vi "Write.vi"(5 "TDMS Channel in":refnum<class "Channel.lvclass">, 8 "error in (no error)":errorcluster, 9 "Channel Properties":refnum<class "Variant.lvclass">, 10 "Array Data":refnum<class "Generic Array Data.lvclass">, 11 "Channel Name":string) -> (0 "error out":errorcluster, 3 "TDMS Channel out":refnum<class "Channel.lvclass">)   [LabVIEW 2020, in "TDMS.lvlib" / "Channel.lvclass"]
doc: "Write Channel Name, Data and Properties."
uses:
  Channel.lvclass
  PPL/HDH.Data.Generic.lvlibp/Generic Data/Generic Array Data/Generic Array Data.lvclass
  PPL/HDH.Data.Generic.lvlibp/Generic Data/Variant/Variant.lvclass
  Channel.lvclass/Channel.ctl
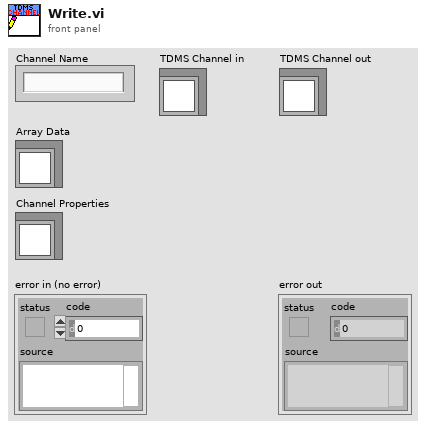
[diagram p1: front panel]
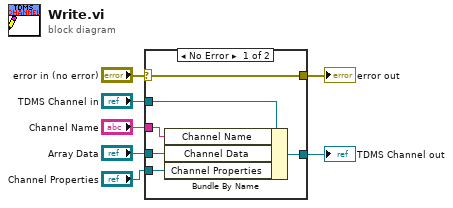
[diagram p0: block diagram]
diagram:
  n1 = case shown="No Error" "error in (no error)" {
    selector: "error in (no error)" -> [w13 w14]
    tunnel: [w13 w14] -> w6
    tunnel: [w11 w15] -> w4
    tunnel: "TDMS Channel in" -> [w12 w15]
    tunnel: "Channel Name" -> [w10 _]
    tunnel: "Array Data" -> [w9 _]
    tunnel: "Channel Properties" -> [w8 _]
    frame No Error {
      n2 = Bundle By Name(cluster=w12, "Channel Name"=w10, "Channel Data"=w9, "Channel Properties"=w8) -> (w11:refnum<class "Channel.lvclass">)
    }
    frame Error {
    }
  }
  "error out" <- w6
  "TDMS Channel out" <- w4
